vi "randomNumber.vi"() -> ()   [LabVIEW 2016]
panel:
  out "x+y":dbl
  in  "y":dbl
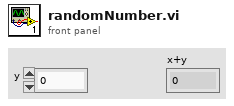
[diagram p1: front panel]
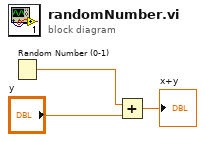
[diagram p0: block diagram]
diagram:
  n1 = Random Number (0-1)() -> (number: 0 to 1=w3:dbl)
  n2 = Add(x=w3, y="y") -> (x+y=→"x+y":dbl)
